vi "Read Group Data.vi"(7 "data type":T1, 8 "error in":errorcluster, 11 "TDMS in":refnum<class "TDMS.lvclass">) -> (0 "error out":errorcluster, 1 "double group data":dbl[][](array[numeric]), 2 "I16 group data":i16[][](array[numeric]), 3 "TDMS out":refnum<class "TDMS.lvclass">, 4 "waveform group data":waveform(dbl)[](array[waveform]), 5 "channel name(s) out":string[](array[string]))   [LabVIEW 2011, in "TDMS.lvclass"]
uses:
  TDMS.lvclass
  Data Type.ctl
  TDMS.lvclass/TDMS.ctl
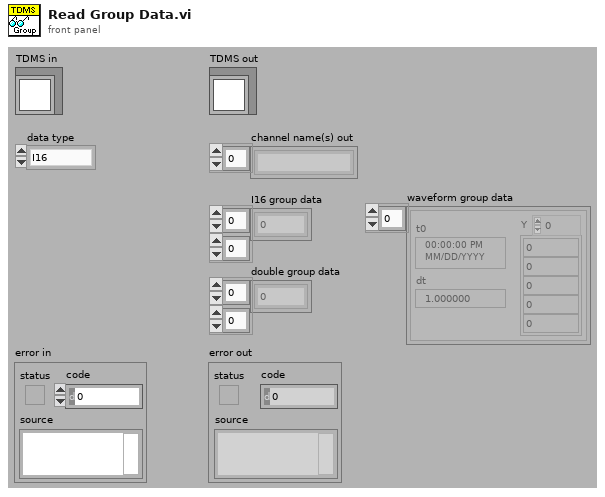
[diagram p1: front panel]
types:
  T1 = typedef "TDMS.lvclass/Data Type.ctl" = enum16{"I16", "Double", "Waveform"}
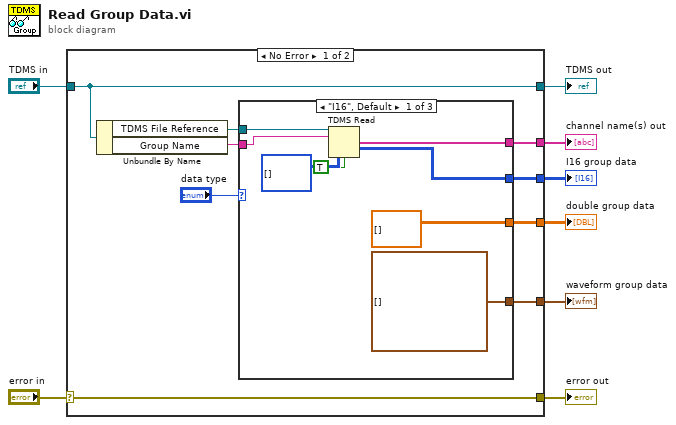
[diagram p0: block diagram]
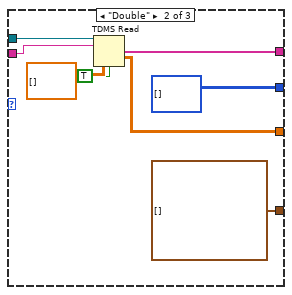
[diagram p2: hidden frame]
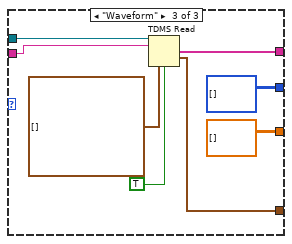
[diagram p3: hidden frame]
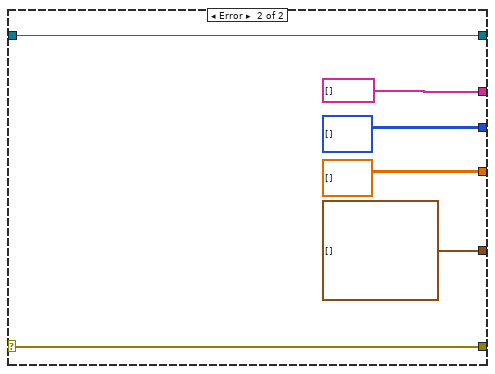
[diagram p4: hidden frame]
diagram:
  n1 = case shown="No Error" "error in" {
    selector: "error in" -> [w17 w47]
    tunnel: [w17 w47] -> w7
    tunnel: [w14 i16[][] [] ("Data Type")] -> w6
    tunnel: [w12 dbl[][] [] ("Data Type")] -> w5
    tunnel: [w11 waveform(dbl)[] []] -> w4
    tunnel: [w10 string[] [] ("channel name(s) out")] -> w3
    tunnel: "TDMS in" -> [w9 w42]
    tunnel: [w9 w42] -> w1
    frame No Error {
      n2 = Unbundle By Name(w9) -> ("TDMS File Reference"=w16:refnum<k34>, "Group Name"=w15:string)
      n3 = case shown="\"I16\", Default" "data type" {
        tunnel: w16 -> [w20 w28 w36]
        tunnel: w15 -> [w19 w27 w35]
        tunnel: [w24 i16[][] [] ("Data Type") i16[][] [] ("Data Type")] -> w14
        tunnel: [dbl[][] [] ("Data Type") w31 dbl[][] [] ("Data Type")] -> w12
        tunnel: [waveform(dbl)[] [] waveform(dbl)[] [] w40] -> w11
        tunnel: [w21 w29 w37] -> w10
        frame "I16", Default {
          n4 = TDMS Read(0:w20, 5:w19, 12:i16[][] [] ("Data Type"), 13:TRUE ("return channels in file order? (F)")) -> (8:w21:string[], 10:w24:i16[][])  [unwired: 4 in, 4 out]
        }
        frame "Double" {
          n5 = TDMS Read(0:w28, 5:w27, 12:dbl[][] [] ("Data Type"), 13:TRUE ("return channels in file order? (F)")) -> (8:w29:string[], 10:w31:dbl[][])  [unwired: 4 in, 4 out]
        }
        frame "Waveform" {
          n6 = TDMS Read(0:w36, 5:w35, 12:waveform(dbl)[] [] ("data type"), 13:TRUE ("return channels in file order? (F)")) -> (8:w37:string[], 10:w40:waveform(dbl)[])  [unwired: 4 in, 4 out]
        }
      }
    }
    frame Error {
    }
  }
  "error out" <- w7
  "I16 group data" <- w6
  "double group data" <- w5
  "waveform group data" <- w4
  "channel name(s) out" <- w3
  "TDMS out" <- w1
